vi "String - Tab (Unicode).vi"() -> (0 "Tab (Unicode)":string)   [LabVIEW 2013]
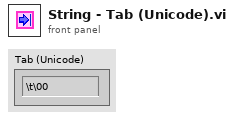
[diagram p1: front panel]
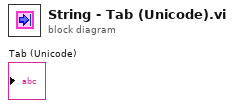
[diagram p0: block diagram]
diagram:
